vi "Get Buffer Size.vi"(0 "phCamera IN":u32, 11 "Error IN":errorcluster) -> (4 "phCamera OUT":u32, 6 "uBufferSize OUT":u32, 8 "uWidth OUT":u32, 10 "uHeight OUT":u32, 14 "uBytesPerPixel OUT":u32, 15 "Error OUT":errorcluster)   [LabVIEW 2014]
uses:
  <vilib>/addons/PixeLINK/Low Level Functions/CAMERA_FEATURES.llb/TDPU-CameraFeatures-FeatureIds.ctl
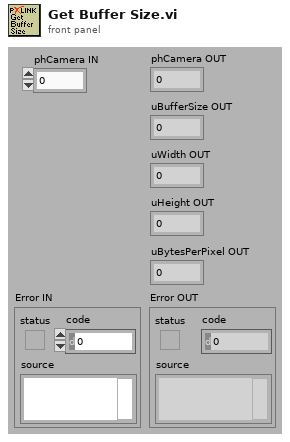
[diagram p1: front panel]
types:
  T1 = typedef "TDPU-CameraFeatures-FeatureIds.ctl" = u32
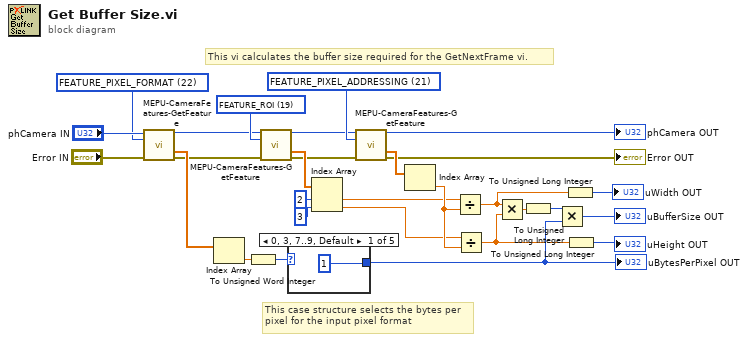
[diagram p0: block diagram]
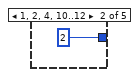
[diagram p2: hidden frame]
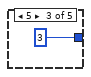
[diagram p3: hidden frame]
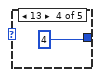
[diagram p4: hidden frame]
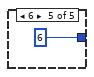
[diagram p5: hidden frame]
diagram:
  w9 = T1 22 items=["FEATURE_BRIGHTNESS", "FEATURE_EXPOSURE", "FEATURE_SHARPNESS", "FEATURE_WHITE_BAL", "FEATURE_HUE", "FEATURE_SATURATION", "FEATURE_GAMMA", "FEATURE_SHUTTER", "FEATURE_GAIN", "FEATURE_IRIS", "FEATURE_FOCUS", "FEATURE_TEMPERATURE", "FEATURE_TRIGGER", "FEATURE_ZOOM", "FEATURE_PAN", "FEATURE_TILT", "FEATURE_OPT_FILTER", "FEATURE_GPIO", "FEATURE_FRAME_RATE", "FEATURE_ROI", "FEATURE_FLIP", "FEATURE_PIXEL_ADDRESSING", "FEATURE_PIXEL_FORMAT", "FEATURE_EXTENDED_SHUTTER", "FEATURE_AUTO_ROI", "FEATURE_LOOKUP_TABLE", "FEATURE_MEMORY_CHANNEL", "FEATURE_WHITE_SHADING", "FEATURE_ROTATE", "FEATURE_IMAGER_CLK_DIVISOR"] ("FEATURE_IDS")
  w17 = T1 21 items=["FEATURE_BRIGHTNESS", "FEATURE_EXPOSURE", "FEATURE_SHARPNESS", "FEATURE_WHITE_BAL", "FEATURE_HUE", "FEATURE_SATURATION", "FEATURE_GAMMA", "FEATURE_SHUTTER", "FEATURE_GAIN", "FEATURE_IRIS", "FEATURE_FOCUS", "FEATURE_TEMPERATURE", "FEATURE_TRIGGER", "FEATURE_ZOOM", "FEATURE_PAN", "FEATURE_TILT", "FEATURE_OPT_FILTER", "FEATURE_GPIO", "FEATURE_FRAME_RATE", "FEATURE_ROI", "FEATURE_FLIP", "FEATURE_PIXEL_ADDRESSING", "FEATURE_PIXEL_FORMAT", "FEATURE_EXTENDED_SHUTTER", "FEATURE_AUTO_ROI", "FEATURE_LOOKUP_TABLE", "FEATURE_MEMORY_CHANNEL", "FEATURE_WHITE_SHADING", "FEATURE_ROTATE", "FEATURE_IMAGER_CLK_DIVISOR"] ("FEATURE_IDS")
  w16 = T1 19 items=["FEATURE_BRIGHTNESS", "FEATURE_EXPOSURE", "FEATURE_SHARPNESS", "FEATURE_WHITE_BAL", "FEATURE_HUE", "FEATURE_SATURATION", "FEATURE_GAMMA", "FEATURE_SHUTTER", "FEATURE_GAIN", "FEATURE_IRIS", "FEATURE_FOCUS", "FEATURE_TEMPERATURE", "FEATURE_TRIGGER", "FEATURE_ZOOM", "FEATURE_PAN", "FEATURE_TILT", "FEATURE_OPT_FILTER", "FEATURE_GPIO", "FEATURE_FRAME_RATE", "FEATURE_ROI", "FEATURE_FLIP", "FEATURE_DECIMATION", "FEATURE_PIXEL_FORMAT", "FEATURE_EXTENDED_SHUTTER", "FEATURE_AUTO_ROI", "FEATURE_LOOKUP_TABLE", "FEATURE_MEMORY_CHANNEL", "FEATURE_ALL"] ("uFeatureId IN")
  # "This case structure selects the bytes per\npixel for the input pixel format"
  # "This vi calculates the buffer size required for the GetNextFrame vi."
  n1 = call <vilib>:"MEPU-CameraFeatures-GetFeature.vi"("hCamera IN"="phCamera IN", "uFeatureId IN"=w9, "Error IN"="Error IN") -> ("hCamera OUT"=w11:u32, "pParms OUT"=w23:dbl[], "Error OUT"=w10:errorcluster)  [unwired: 8 in, 2 out]
  n2 = Index Array(array=w23) -> (element=w24:dbl)  [unwired: 1 in]
  n3 = To Unsigned Word Integer(number=w24) -> (unsigned 16bit integer=w25:u16)
  n4 = call <vilib>:"MEPU-CameraFeatures-GetFeature.vi"("hCamera IN"=w11, "uFeatureId IN"=w16, "Error IN"=w10) -> ("hCamera OUT"=w15:u32, "pParms OUT"=w20:dbl[], "Error OUT"=w14:errorcluster)  [unwired: 8 in, 2 out]
  n5 = case shown="0, 3, 7..9, Default" w25 {
    tunnel: [u32 1 u32 2 u32 3 u32 4 u32 6] -> w26
    frame 0, 3, 7..9, Default {
    }
    frame 1, 2, 4, 10..12 {
    }
    frame 5 {
    }
    frame 13 {
    }
    frame 6 {
    }
  }
  "uBytesPerPixel OUT" <- w26
  n6 = Index Array(array=w20, index #1=2 ("index"), index #2=3 ("index")) -> (element #1=w6:dbl, element #2=w5:dbl)
  n7 = call <vilib>:"MEPU-CameraFeatures-GetFeature.vi"("hCamera IN"=w15, "uFeatureId IN"=w17, "Error IN"=w14) -> ("hCamera OUT"=→"phCamera OUT":u32, "pParms OUT"=w21:dbl[], "Error OUT"=→"Error OUT":errorcluster)  [unwired: 8 in, 2 out]
  n8 = Index Array(array=w21) -> (element=w22:dbl)  [unwired: 1 in]
  n9 = Divide(x=w6, y=w22) -> (x/y=w2:dbl)
  n10 = Divide(x=w5, y=w22) -> (x/y=w1:dbl)
  n11 = Multiply(x=w2, y=w1) -> (x*y=w27:dbl)
  n12 = To Unsigned Long Integer(number=w27) -> (unsigned 32bit integer=w28:u32)
  n13 = Multiply(x=w28, y=w26) -> (x*y=→"uBufferSize OUT":u32)
  n14 = To Unsigned Long Integer(number=w2) -> (unsigned 32bit integer=→"uWidth OUT":u32)
  n15 = To Unsigned Long Integer(number=w1) -> (unsigned 32bit integer=→"uHeight OUT":u32)
